vi "Plant System.vi"(1 "积分器？":bool, 2 "输出饱和范围":cluster{"输出上限":dbl, "输出下限":dbl}={"输出上限"=inf, "输出下限"=-inf}, 7 "设备输入":dbl format="%.2f", 11 "dt (s)":dbl=-1.0 format="%.3f", 12 "重新初始化？(F)":bool, 13 "过程参数":T1={"静态增益"=2.5, "滞后(s)"=2.5, "死区时间(s)"=0.001, "加载"=0.0, "死区"=0.0, "传感器噪声"=0.0, "初始PV"=30.0, "设备噪声"=0.0} {"设备噪声" format="%.2f"; "初始PV" format="%.2f"; "传感器噪声" format="%.2f"; "滞后(s)" format="%.2f"; "死区时间(s)" format="%.2f"; "死区" format="%.1f"; "加载" format="%.2f"; "静态增益" format="%.2f"}) -> (8 "设备输出":dbl format="%.2f")   [LabVIEW 2016]
doc: "仿真物理设备响应；与反馈控制回路配合使用。\n\n所有刻度单位均为百分比。滞后时间单位为分。过程死区时间为真死区时间，作为多循环周期时间来衡量。注意：该死区时间取决于VI调用的间隔。可以修改该处使用的算法，来仿真任意过程。\n\n如果同时需要仿真多个设备，则用不同文件名保存该VI副本。"
uses:
  <vilib>/addons/control/pid/pid.llb/PID Lead-Lag (DBL).vi
  <vilib>/addons/control/pid/NI_PID_pid.lvlib
  <vilib>/addons/control/advanced/NI_AdvCtrl_nonlinear.lvlib
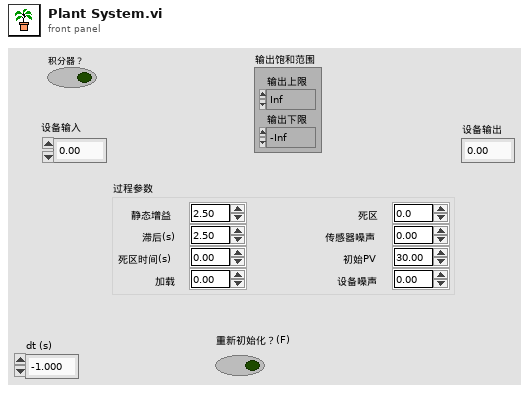
[diagram p1: front panel]
types:
  T1 = cluster{"静态增益":dbl, "滞后(s)":dbl, "死区时间(s)":dbl, "加载":dbl, "死区":dbl, "传感器噪声":dbl, "初始PV":dbl, "设备噪声":dbl}
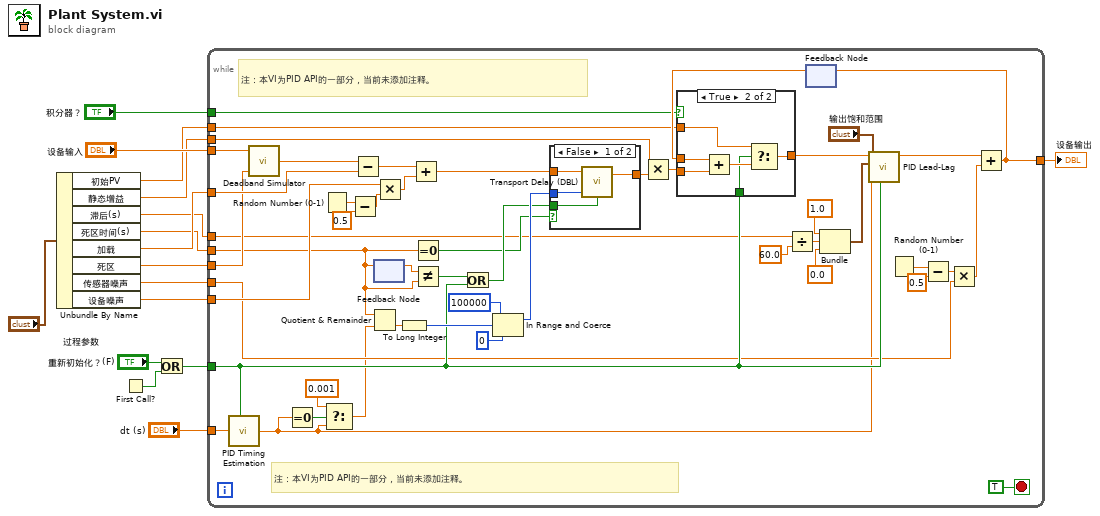
[diagram p0: block diagram]
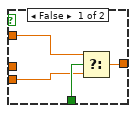
[diagram p3: hidden frame]
diagram:
  n1 = Unbundle By Name("过程参数") -> ("初始PV"=w1:dbl, "静态增益"=w5:dbl, "滞后(s)"=w3:dbl, "死区时间(s)"=w6:dbl, "加载"=w9:dbl, "死区"=w8:dbl, "传感器噪声"=w2:dbl, "设备噪声"=w10:dbl)
  n2 = First Call?() -> (First Call?: T/F=w15:bool)
  n3 = Or(x="重新初始化？(F)", y=w15) -> (x .or. y?=w14:bool)
  n4 = while {
    tunnel: w14 -> [w32]
    tunnel: "dt (s)" -> [w33]
    tunnel: [w49] -> w12
    tunnel: w10 -> [w30]
    tunnel: w9 -> [w29]
    tunnel: w8 -> [w28]
    tunnel: "设备输入" -> [w27]
    tunnel: w6 -> [w20]
    tunnel: w5 -> [w26]
    tunnel: "积分器？" -> [w25]
    tunnel: w3 -> [w17]
    tunnel: w2 -> [w24]
    tunnel: w1 -> [w18]
    stop <- TRUE stop-if-true
    # "注：本VI为PID API的一部分，当前未添加注释。"
    # "注：本VI为PID API的一部分，当前未添加注释。"
    n5 = call <vilib>:"PID Timing Estimation.vi"("Initialize?"=w32, "dt (s) in"=w33) -> ("dt (s) out"=w23:dbl)  [unwired: 7 in]
    n6 = call "Deadband Simulator.vi"("死区(%)"=w28, "请求位置(%)"=w27) -> ("实际位置(%)"=w45:dbl)  [unwired: 1 in]
    n7 = Equal To 0?(x=w23) -> (x = 0?=w35:bool)
    n8 = Random Number (0-1)() -> (number: 0 to 1=w63:dbl)
    n9 = Select(t=0.001, s=w35, f=w23) -> (s? t:f=w21:dbl)
    n10 = Subtract(x=w63, y=0.5) -> (x-y=w31:dbl)
    n11 = Subtract(x=w45, y=w29) -> (x-y=w44:dbl)
    n12 = Quotient & Remainder(x=w20, y=w21) -> (floor(x/y)=w51:dbl)  [unwired: 1 out]
    n13 = feedback-in #1(w20) -> ()
    n14 = feedback #1() -> (w41:dbl)  [unwired: 1 in]
    n15 = Multiply(x=w30, y=w31) -> (x*y=w65:dbl)
    n16 = To Long Integer(number=w51) -> (32bit integer=w39:i32)
    n17 = Add(x=w44, y=w65) -> (x+y=w43:dbl)
    n18 = Equal To 0?(x=w20) -> (x = 0?=w19:bool)
    n19 = Not Equal?(x=w41, y=w20) -> (x != y?=w40:bool)
    n20 = Or(x=w40, y=w32) -> (x .or. y?=w22:bool)
    n21 = In Range and Coerce(upper limit=100000, x=w39, lower limit=0) -> (coerced(x)=w36:i32)  [unwired: 1 out]
    n22 = case shown="False" w19 {
      tunnel: [w69 w70] -> w50
      tunnel: w43 -> [w68 w70]
      tunnel: w36 -> [w67 _]
      tunnel: w22 -> [w66 _]
      frame False {
        n23 = call <vilib>:"Transport Delay (DBL).vi"("initialize"=w66, "delay"=w67, "input point"=w68) -> ("output point"=w69:dbl)  [unwired: 2 in]
      }
      frame True {
      }
    }
    n24 = Multiply(x=w26, y=w50) -> (x*y=w42:dbl)
    n25 = Divide(x=w17, y=60.0) -> (x/y=w47:dbl)
    n26 = feedback #2() -> (w57:dbl)  [unwired: 1 in]
    n27 = case shown="True" w25 {
      tunnel: w42 -> [w73 w80]
      tunnel: [w72 w78] -> w60
      tunnel: w18 -> [w71 w77]
      tunnel: w57 -> [_ w76]
      tunnel: w32 -> [w74 w75]
      frame False {
        n28 = Select(t=w71, s=w74, f=w73) -> (s? t:f=w72:dbl)
      }
      frame True {
        n29 = Add(x=w76, y=w80) -> (x+y=w79:dbl)
        n30 = Select(t=w77, s=w75, f=w79) -> (s? t:f=w78:dbl)
      }
    }
    n31 = Bundle(1.0, w47, 0.0) -> (w58:cluster{dbl, dbl, dbl})  [unwired: 1 in]
    n32 = call-poly <vilib>:"PID Lead-Lag.vi"("reinitialize? (F)"=w32, "dt (s)"=w23, "output range"="输出饱和范围", "tuning parameters"=w58, "input"=w60) -> ("output"=w53:dbl)  [unwired: 3 in, 1 out]
    n33 = Random Number (0-1)() -> (number: 0 to 1=w56:dbl)
    n34 = Subtract(x=w56, y=0.5) -> (x-y=w55:dbl)
    n35 = Multiply(x=w55, y=w24) -> (x*y=w52:dbl)
    n36 = Add(x=w53, y=w52) -> (x+y=w49:dbl)
    n37 = feedback-in #2(w49) -> ()
  }
  "设备输出" <- w12
